vi "PCO_SetBitAlignment.vi"(8 "error in (no error)":errorcluster {"code" format="%x"}, 10 "wBitAlignment":u16(ring) items=["BIT_ALIGNMENT_MSB", "BIT_ALIGNMENT_LSB"], 11 "ph":u64) -> (0 "error out":errorcluster {"code" format="%x"}, 2 "ErrorMessage":i32 format="%x", 3 "ph out":u64)   [LabVIEW 2019, in "SDK.lvlib" / "ImageInformation.lvlib"]
doc: "<b>Description:</b>\nThis function does set the current bit alignment of the transferred image data.\nSee PCO_GetBitAlignment for further details.\n\n<b>Supported camera type:</b>\nAll cameras\n\n<b>Descriptor dependency:</b>\nNone"
uses:
  ImageInformation.lvlib
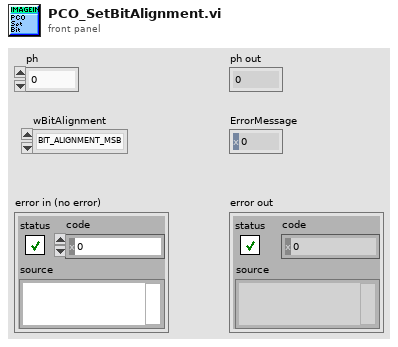
[diagram p1: front panel]
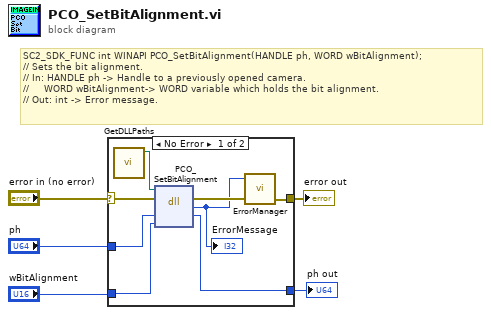
[diagram p0: block diagram]
diagram:
  # "SC2_SDK_FUNC int WINAPI PCO_SetBitAlignment(HANDLE ph, WORD wBitAlignment);\n// Sets the bit alignment.\n// In: HANDLE ph -> Handle to a previously opened camera.\n//     WORD wBitAlignment-> WORD variable which holds the bit alignment.\n// Out: int -> Error message."
  n1 = case shown="No Error" "error in (no error)" {
    selector: "error in (no error)" -> [w11 w15]
    tunnel: "ph" -> [w13 w14]
    tunnel: [w12 w14] -> w4
    tunnel: "wBitAlignment" -> [w7 _]
    tunnel: [w9 w15] -> w2
    frame No Error {
      n2 = call "GetDLLPaths.vi"() -> ("SC2_Cam_Path"=w6:path)  [unwired: 9 in, 2 out]
      n3 = dll-call lib="?" fn="PCO_SetBitAlignment"(path in=w6, error in=w11, "ph"=w13, "wBitAlignment"=w7) -> (error out=w10:errorcluster, "return type"=w8:i32, "ph"=w12:u64)  [unwired: 2 in, 1 out]
      "ErrorMessage" <- w8
      n4 = call "ErrorManager.vi"("error in (no error)"=w10, "error code"=w8) -> ("error out"=w9:errorcluster)  [unwired: 3 in]
    }
    frame Error {
    }
  }
  "ph out" <- w4
  "error out" <- w2
